vi "Find Open Neighbor.vi"(9 "X":i32, 10 "Y":i32, 11 "our positions":u8[][](array[numeric])) -> (0 "open count":i16, 1 "open?":bool, 2 "open y":i32, 3 "open x":i32, 4 "open direction":T1, 6 "friendly zone":bool)   [LabVIEW 2020, in "Uno.lvclass"]
uses:
  Uno.lvclass
  Type Defs/Direction Enum.ctl
  Type Defs/SB Type Defs.lvlib
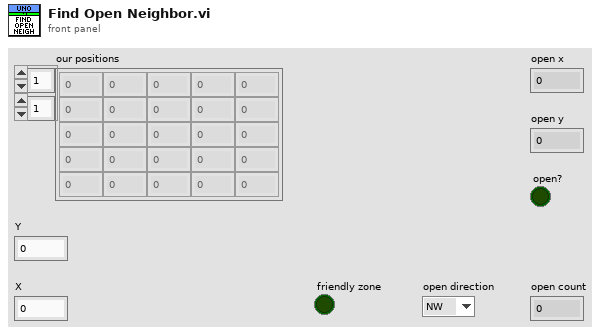
[diagram p1: front panel]
types:
  T1 = typedef "SB Type Defs.lvlib/Direction Enum.ctl" = enum16{"NW", "N", "NE", "E", "SE", "S", "SW", "W"}
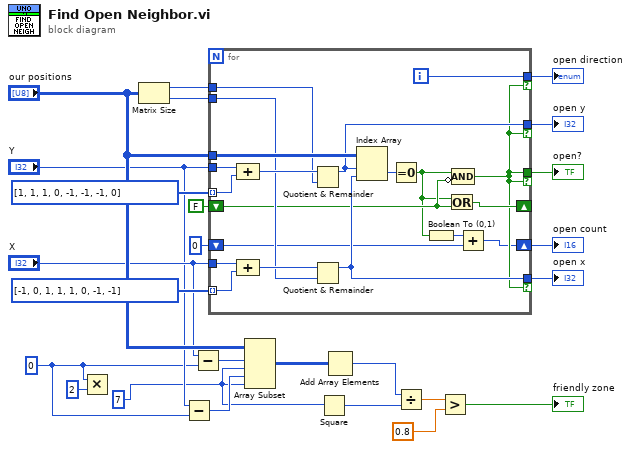
[diagram p0: block diagram]
diagram:
  w1 = 7 ("y")
  w8 = 0 ("y")
  n1 = Multiply(x=w8, y=2) -> ()  [unwired: 1 out]
  n2 = Matrix Size(0:"our positions") -> (1:w19:i32, 2:w20:i32)
  n3 = Subtract(x="Y", y=w8) -> (x-y=w10:i32)
  n4 = Subtract(x="X", y=w8) -> (x-y=w13:i32)
  n5 = for {
    tunnel: "our positions" -> [w45]
    tunnel: w19 -> [w41]
    tunnel: w20 -> [w42]
    tunnel: "X" -> [w40]
    tunnel: "Y" -> [w39]
    tunnel: [w30] -> w18 if=w30
    tunnel: [w38] -> w21 if=w30
    tunnel: [w34] -> w22 if=w30
    tunnel: [w35] -> w23 if=w30
    tunnel: i32[] [1, 1, 1, 0, -1, -1, -1, 0] -> [w37] mode=indexing
    tunnel: i32[] [-1, 0, 1, 1, 1, 0, -1, -1] -> [w36] mode=indexing
    shift-right: [w32] -> _
    shift-left: FALSE -> [w31]
    shift-right: [w27] -> w16
    shift-left: i16 0 -> [w26]
    i -> [w38]
    n6 = Compound Arithmetic op=ADD(w39, w37) -> (w43:i32)
    n7 = Compound Arithmetic op=ADD(w40, w36) -> (w44:i32)
    n8 = Quotient & Remainder(x=w43, y=w41) -> (x-y*floor(x/y)=w34:i32)  [unwired: 1 out]
    n9 = Quotient & Remainder(x=w44, y=w42) -> (x-y*floor(x/y)=w35:i32)  [unwired: 1 out]
    n10 = Index Array(array=w45, index (row)=w34, index (col)=w35) -> (element=w33:u8)
    n11 = Equal To 0?(x=w33) -> (x = 0?=w29:bool)
    n12 = Boolean To (0,1)(Boolean=w29) -> (0, 1=w28:i16)
    n13 = Or(x=w29, y=w31) -> (x .or. y?=w32:bool)
    n14 = Compound Arithmetic op=AND(w29, invert w31) -> (w30:bool)
    n15 = Add(x=w28, y=w26) -> (x+y=w27:i16)
  }
  "open x" <- w23
  "open y" <- w22
  "open direction" <- w21
  "open?" <- w18
  "open count" <- w16
  n16 = Array Subset(array="our positions", index (row)=w13, length (row)=w1, index (col)=w10, length (col)=w1) -> (w7:u8[][])
  n17 = Square(x=w1) -> (x^2=w5:i32)
  n18 = Add Array Elements(numeric array=w7) -> (sum=w6:u8)
  n19 = Divide(x=w6, y=w5) -> (x/y=w4:dbl)
  n20 = Greater?(x=w4, y=0.8) -> (0:→"friendly zone":bool)
